vi "PreObjectInitialize.vi"(8 "error in (no error)":errorcluster, 11 "AFM.Asylum in":refnum<class "Asylum_Driver.lvclass">) -> (0 "error out":errorcluster, 3 "AFM.Asylum out":refnum<class "Asylum_Driver.lvclass">)   [LabVIEW 2019, in "Asylum_Driver.lvclass"]
uses:
  Asylum_Driver.lvclass
  AFM Driver/AFM_Driver.lvclass
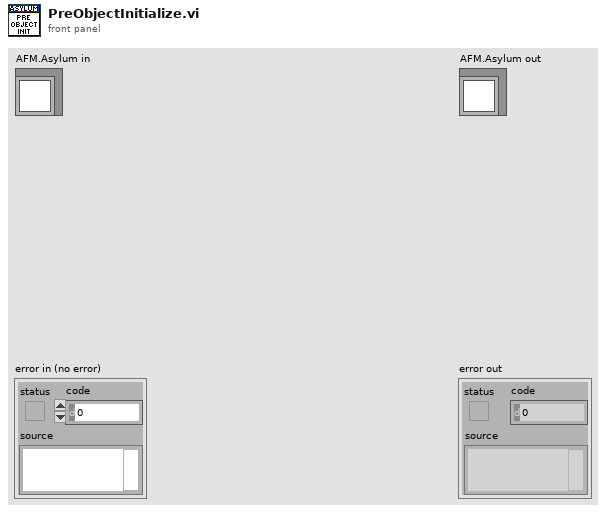
[diagram p1: front panel]
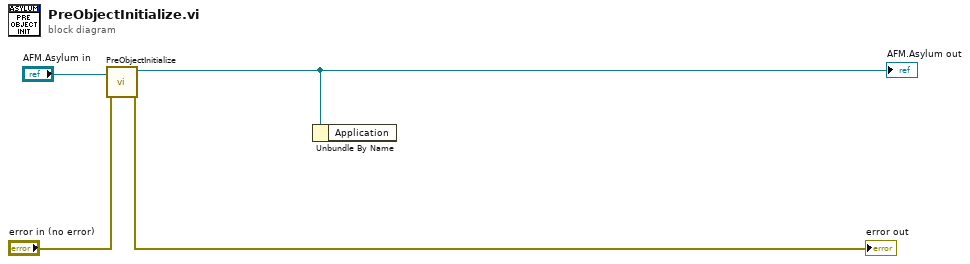
[diagram p0: block diagram]
diagram:
  n1 = call-parent "PreObjectInitialize.vi"("error in (no error)"="error in (no error)", "AFM.Asylum in"="AFM.Asylum in") -> ("error out"=→"error out":errorcluster, "AFM.Asylum out"=w1:refnum<class "Asylum_Driver.lvclass">)  [unwired: 8 in]
  "AFM.Asylum out" <- w1
  n2 = Unbundle By Name(w1) -> ()  [unwired: 1 out]
